vi "FMA1600A General Setup.vi"(5 "Gas Type":T2, 6 "baud rate (19200)":u32=19200, 7 "Unit ID":string, 8 "error in (no error)":errorcluster, 10 "Set STP Register":bool, 11 "VISA Refnum in":refnum<visa-resource-name>) -> (0 "error out":errorcluster, 2 "Measurement Units":T1, 3 "VISA Refnum out":refnum<visa-resource-name>)   [LabVIEW 2018]
uses:
  Type Definitions/FMA1600A Gas Type.ctl
  Type Definitions/FMA1600A Units String.ctl
  Type Definitions/FMA1600A Commands.ctl
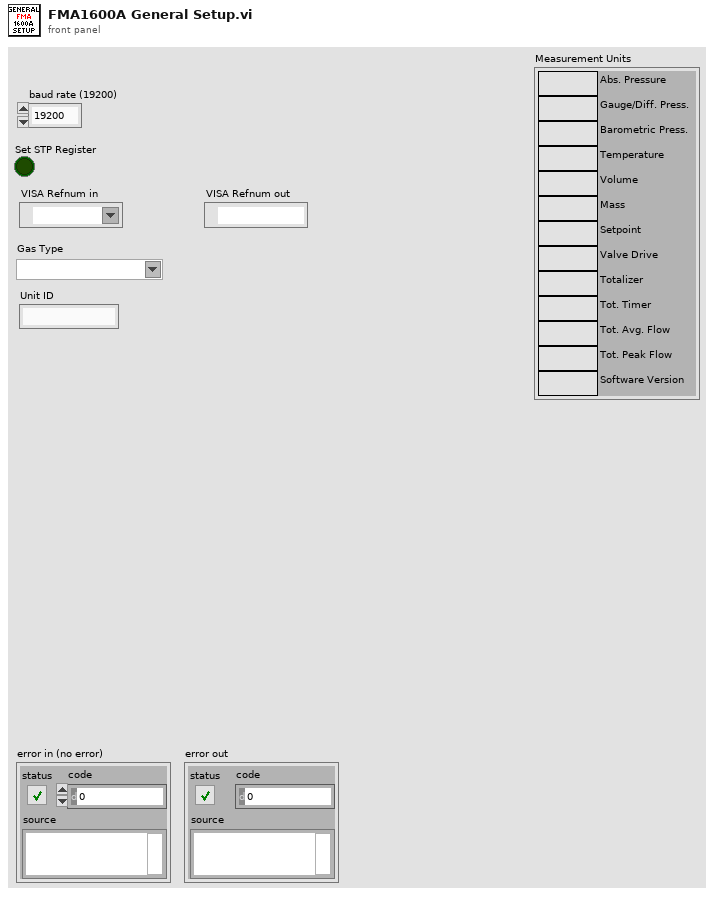
[diagram p1: front panel]
types:
  T1 = typedef "FMA1600A Units String.ctl" = cluster{"Abs. Pressure":string, "Gauge/Diff. Press.":string, "Barometric Press.":string, "Temperature":string, "Volume":string, "Mass":string, "Setpoint":string, "Valve Drive":string, "Totalizer":string, "Tot. Timer":string, "Tot. Avg. Flow":string, "Tot. Peak Flow":string, "Software Version":string}
  T2 = typedef "FMA1600A Gas Type.ctl" = string
  T3 = typedef "FMA1600A Commands.ctl" = string
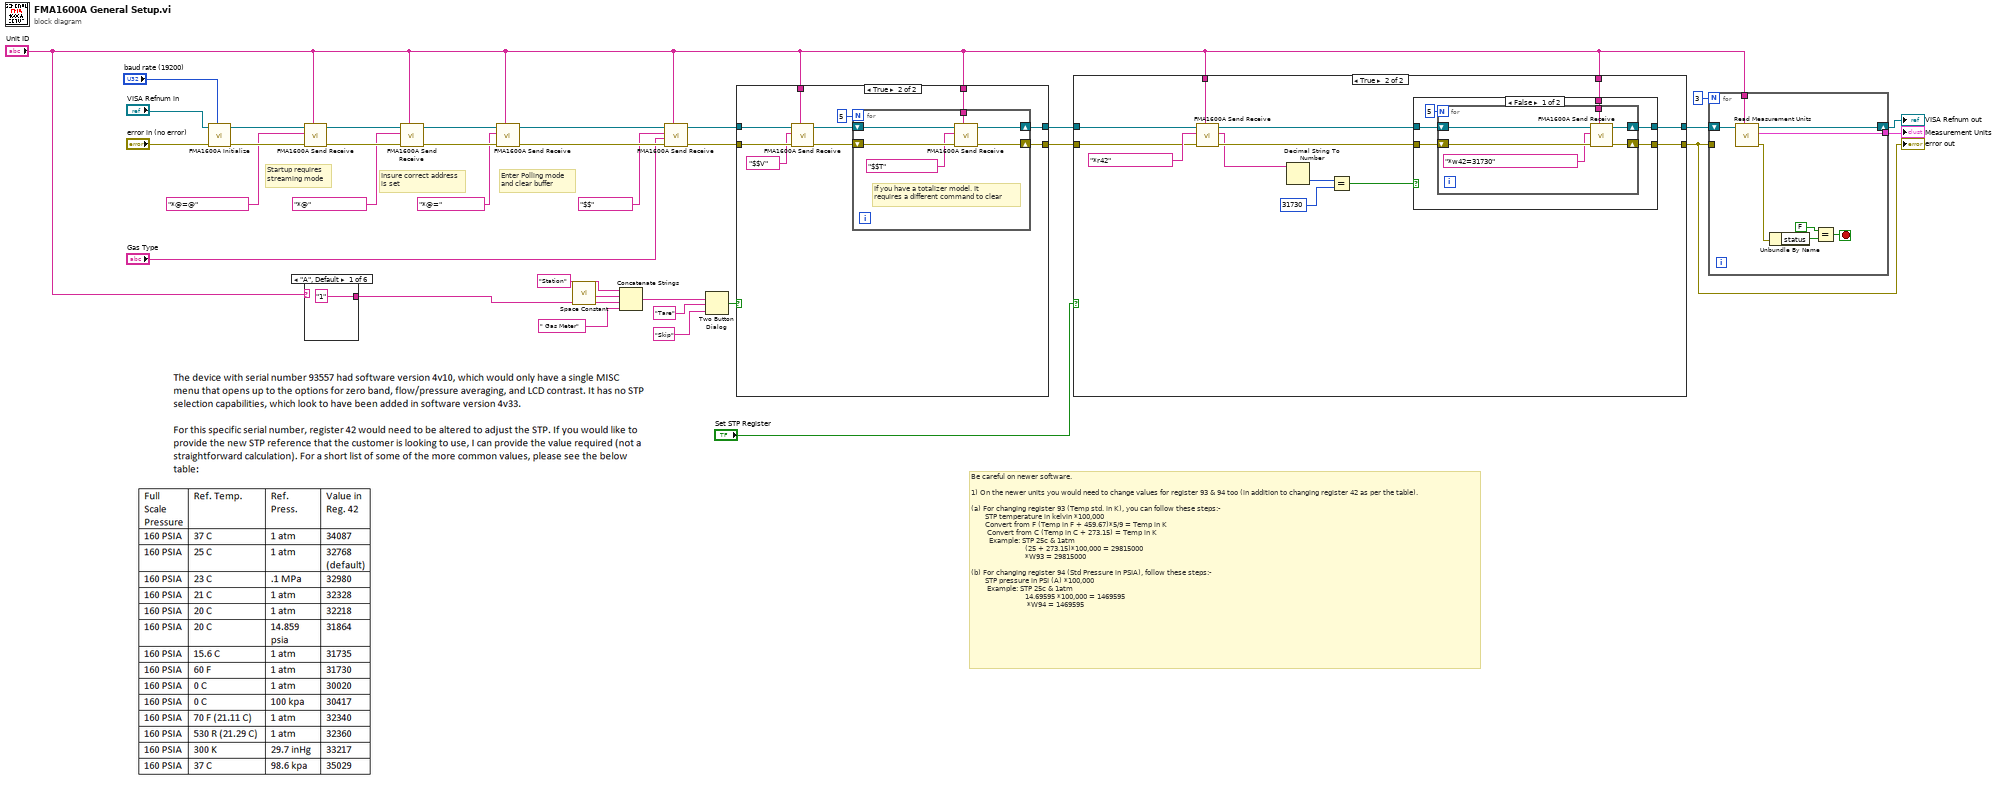
[diagram p0: block diagram]
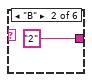
[diagram p4: hidden frame]
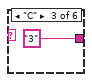
[diagram p5: hidden frame]
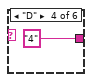
[diagram p6: hidden frame]
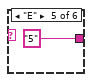
[diagram p7: hidden frame]
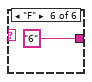
[diagram p8: hidden frame]
diagram:
  # "Be careful on newer software.\n\n1) On the newer units you would need to change values for register 93 & 94 too (in addition to changing register 42 as per the table). \n\n(a) For changing register 93 (Temp std. in K), you can follow these steps:-\n       STP temperature in kelvin *100,000\n       Convert from F (Temp in F + 459.67)*5/9 = Temp in K\n        Convert from C (Temp in C + 273.15) = Temp in K\n         Example: STP 25c & 1atm\n                           (25 + 273.15)*100,000 = 29815000\n                           *W93 = 29815000\n\n(b) For changing register 94 (Std Pressure in PSIA), follow these steps:-\n       STP pressure in PSI (A) *100,000\n        Example: STP 25c & 1atm\n                           14.69595 *100,000 = 1469595\n                            *W94 = 1469595"
  # "Startup requires \nstreaming mode"
  # "Insure correct address\nis set"
  # "Enter Polling mode\nand clear buffer"
  n1 = call "FMA1600A Initialize.vi"("baud rate (9600)"="baud rate (19200)", "error in (no error)"="error in (no error)", "VISA Refnum in"="VISA Refnum in") -> ("error out"=w30:errorcluster, "VISA Refnum out"=w31:refnum<visa-resource-name>)  [unwired: 7 in]
  n2 = call "FMA1600A Send Receive.vi"("Unit ID"="Unit ID", "error in (no error)"=w30, "FMA1600A Commands"=T3 "*@=@", "VISA Refnum in"=w31) -> ("error out"=w32:errorcluster, "VISA Refnum out"=w33:refnum<visa-resource-name>)  [unwired: 5 in, 1 out]
  n3 = case shown="\"A\", Default" "Unit ID" {
    tunnel: ["1" ("message") "2" ("message") "3" ("message") "4" ("message") "5" ("message") "6" ("message")] -> w20
    frame "A", Default {
    }
    frame "B" {
    }
    frame "C" {
    }
    frame "D" {
    }
    frame "E" {
    }
    frame "F" {
    }
  }
  n4 = call "FMA1600A Send Receive.vi"("Unit ID"="Unit ID", "error in (no error)"=w32, "FMA1600A Commands"=T3 "*@", "VISA Refnum in"=w33) -> ("error out"=w35:errorcluster, "VISA Refnum out"=w34:refnum<visa-resource-name>)  [unwired: 5 in, 1 out]
  n5 = call "FMA1600A Send Receive.vi"("Unit ID"="Unit ID", "error in (no error)"=w35, "FMA1600A Commands"=T3 "*@=", "VISA Refnum in"=w34) -> ("error out"=w27:errorcluster, "VISA Refnum out"=w24:refnum<visa-resource-name>)  [unwired: 5 in, 1 out]
  n6 = call <vilib>:"Space Constant.vi"() -> ("String"=w7:string)
  n7 = Concatenate Strings("Station" ("message"), w7, w20, " Gas Meter" ("string")) -> (w11:string)
  n8 = call "FMA1600A Send Receive.vi"("Unit ID"="Unit ID", "error in (no error)"=w27, "Gas Type"="Gas Type", "FMA1600A Commands"=T3 "$$", "VISA Refnum in"=w24) -> ("error out"=w26:errorcluster, "VISA Refnum out"=w25:refnum<visa-resource-name>)  [unwired: 4 in, 1 out]
  n9 = Two Button Dialog(message=w11, 1:"Skip" ("F button name (\"Cancel\")"), 2:"Tare" ("T button name (\"OK\")")) -> (T button?=w22:bool)
  n10 = case shown="True" w22 {
    tunnel: [w42 w47] -> w12
    tunnel: [w43 w46] -> w13
    tunnel: w26 -> [w43 w53]
    tunnel: w25 -> [w42 w52]
    tunnel: "Unit ID" -> [_ w51]
    tunnel: "Unit ID" -> [_ w45]
    frame False {
    }
    frame True {
      n11 = call "FMA1600A Send Receive.vi"("Unit ID"=w51, "error in (no error)"=w53, "FMA1600A Commands"=T3 "$$V", "VISA Refnum in"=w52) -> ("error out"=w49:errorcluster, "VISA Refnum out"=w48:refnum<visa-resource-name>)  [unwired: 5 in, 1 out]
      n12 = for {
        N: 5 -> [_]
        tunnel: w45 -> [w55]
        shift-right: [w56] -> w46
        shift-left: w49 -> [w59]
        shift-right: [w57] -> w47
        shift-left: w48 -> [w58]
        # "If you have a totalizer model. It \nrequires a different command to clear"
        n13 = call "FMA1600A Send Receive.vi"("Unit ID"=w55, "error in (no error)"=w59, "FMA1600A Commands"=T3 "$$T", "VISA Refnum in"=w58) -> ("error out"=w56:errorcluster, "VISA Refnum out"=w57:refnum<visa-resource-name>)  [unwired: 5 in, 1 out]
      }
    }
  }
  n14 = case shown="True" "Set STP Register" {
    tunnel: [w60 w74] -> w4
    tunnel: [w61 w73] -> w2
    tunnel: w13 -> [w61 w69]
    tunnel: w12 -> [w60 w70]
    tunnel: "Unit ID" -> [_ w72]
    tunnel: "Unit ID" -> [_ w66]
    frame False {
    }
    frame True {
      n15 = call "FMA1600A Send Receive.vi"("Unit ID"=w66, "error in (no error)"=w69, "FMA1600A Commands"=T3 "*r42", "VISA Refnum in"=w70) -> ("error out"=w67:errorcluster, "Raw FMA1600A Data"=w65:string, "VISA Refnum out"=w68:refnum<visa-resource-name>)  [unwired: 5 in]
      n16 = Decimal String To Number(string=w65) -> (number=w64:i32)  [unwired: 2 in, 1 out]
      n17 = Equal?(x=w64, y=31730) -> (x = y?=w62:bool)
      n18 = case shown="False" w62 {
        tunnel: [w80 w87] -> w74
        tunnel: [w79 w88] -> w73
        tunnel: w72 -> [w78 _]
        tunnel: w68 -> [w76 w87]
        tunnel: w67 -> [w75 w88]
        frame False {
          n19 = for {
            N: 5 -> [_]
            tunnel: w78 -> [w82]
            shift-right: [w85] -> w79
            shift-left: w75 -> [w84]
            shift-right: [w86] -> w80
            shift-left: w76 -> [w83]
            n20 = call "FMA1600A Send Receive.vi"("Unit ID"=w82, "error in (no error)"=w84, "FMA1600A Commands"=T3 "*w42=31730", "VISA Refnum in"=w83) -> ("error out"=w85:errorcluster, "VISA Refnum out"=w86:refnum<visa-resource-name>)  [unwired: 5 in, 1 out]
          }
        }
        frame True {
        }
      }
    }
  }
  "error out" <- w2
  n21 = for {
    N: 3 -> [_]
    tunnel: "Unit ID" -> [w95]
    tunnel: [w93] -> w3
    shift-right: [w96] -> w6
    shift-left: w4 -> [w94]
    tunnel: w2 -> [_]
    stop <- w89 stop-if-true
    n22 = call "Read Measurement Units.vi"("Unit ID (A)"=w95, "VISA Session In"=w94) -> ("error out"=w92:errorcluster, "Measurement Units"=w93:T1, "VISA Session Out"=w96:refnum<visa-resource-name>)  [unwired: 6 in, 1 out]
    n23 = Unbundle By Name(w92) -> ("status"=w91:bool)
    n24 = Equal?(x=FALSE, y=w91) -> (x = y?=w89:bool)
  }
  "VISA Refnum out" <- w6
  "Measurement Units" <- w3
